vi "Read PlatMods.vi"(8 "error in (no error)":errorcluster, 11 "ControlKeyUpMsg in":refnum<class "ControlKeyUpMsg.lvclass">) -> (0 "error out":errorcluster, 2 "PlatMods":T1, 3 "ControlKeyUpMsg out":refnum<class "ControlKeyUpMsg.lvclass">)   [LabVIEW 2017, in "ActorEvents.lvlib" / "ControlKeyUpMsg.lvclass"]
uses:
  ControlKeyUpMsg.lvclass
  ControlKeyUpMsg.lvclass/ControlKeyUpMsg.ctl
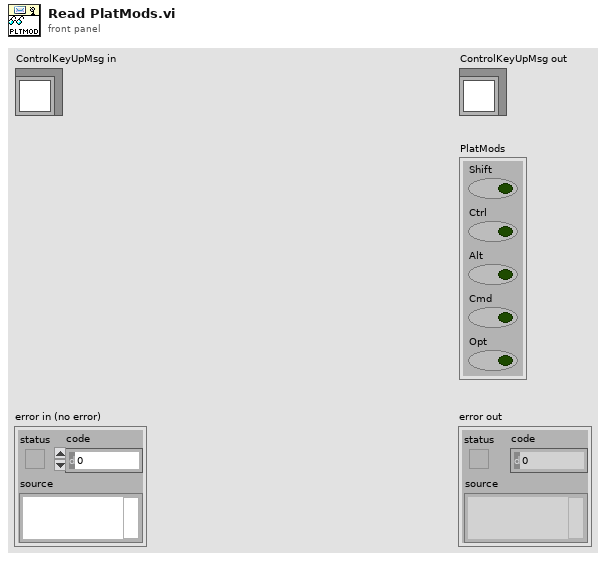
[diagram p1: front panel]
types:
  T1 = cluster{"Shift":bool, "Ctrl":bool, "Alt":bool, "Cmd":bool, "Opt":bool}
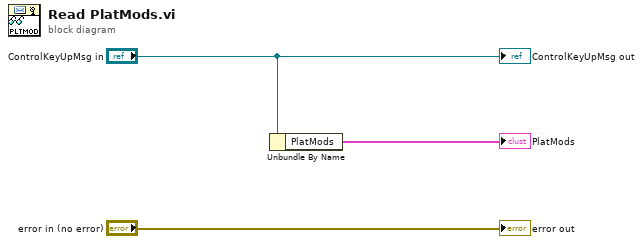
[diagram p0: block diagram]
diagram:
  n1 = Unbundle By Name("ControlKeyUpMsg in") -> ("PlatMods"=→"PlatMods":T1)
  "error out" <- "error in (no error)"
  "ControlKeyUpMsg out" <- "ControlKeyUpMsg in"
